vi "test wait for alive.vi"() -> ()   [LabVIEW 2014]
uses:
  user.lib/_NEVSTOP/Communicable State Machine(CSM)/_Support/Priority Queue/Priority Queue.lvclass/Priority Queue.ctl
  user.lib/_NEVSTOP/Communicable State Machine(CSM)/Utility/uuid.vi
  user.lib/_NEVSTOP/Communicable State Machine(CSM)/_Support/Process/CSMP-Async Call.vi
  user.lib/_NEVSTOP/Communicable State Machine(CSM)/Utility/Trim Both Whitespace.vi
  user.lib/_NEVSTOP/Communicable State Machine(CSM)/_Support/CSMQ/_CSMObj-Message Check.vi
  user.lib/_NEVSTOP/Communicable State Machine(CSM)/_Support/CSMQ/_CSMObj-Enqueue Cross-Module Message.vi
  user.lib/_NEVSTOP/Communicable State Machine(CSM)/_Support/CSMQ/_CSMOFGV Get.vi
  user.lib/_NEVSTOP/Communicable State Machine(CSM)/_Support/Priority Queue/Enqueue Element.vi
  user.lib/_NEVSTOP/Communicable State Machine(CSM)/Utility/Build Error Cluster.vi
  user.lib/_NEVSTOP/Communicable State Machine(CSM)/_Support/CSMQ/_CSMOFGV.vi
  user.lib/_NEVSTOP/Communicable State Machine(CSM)/Communicable State Machine.lvlib
panel:
  out "waited(ms) 2":u32
  out "waited(ms)":u32
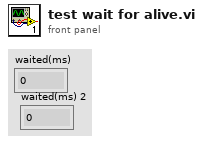
[diagram p1: front panel]
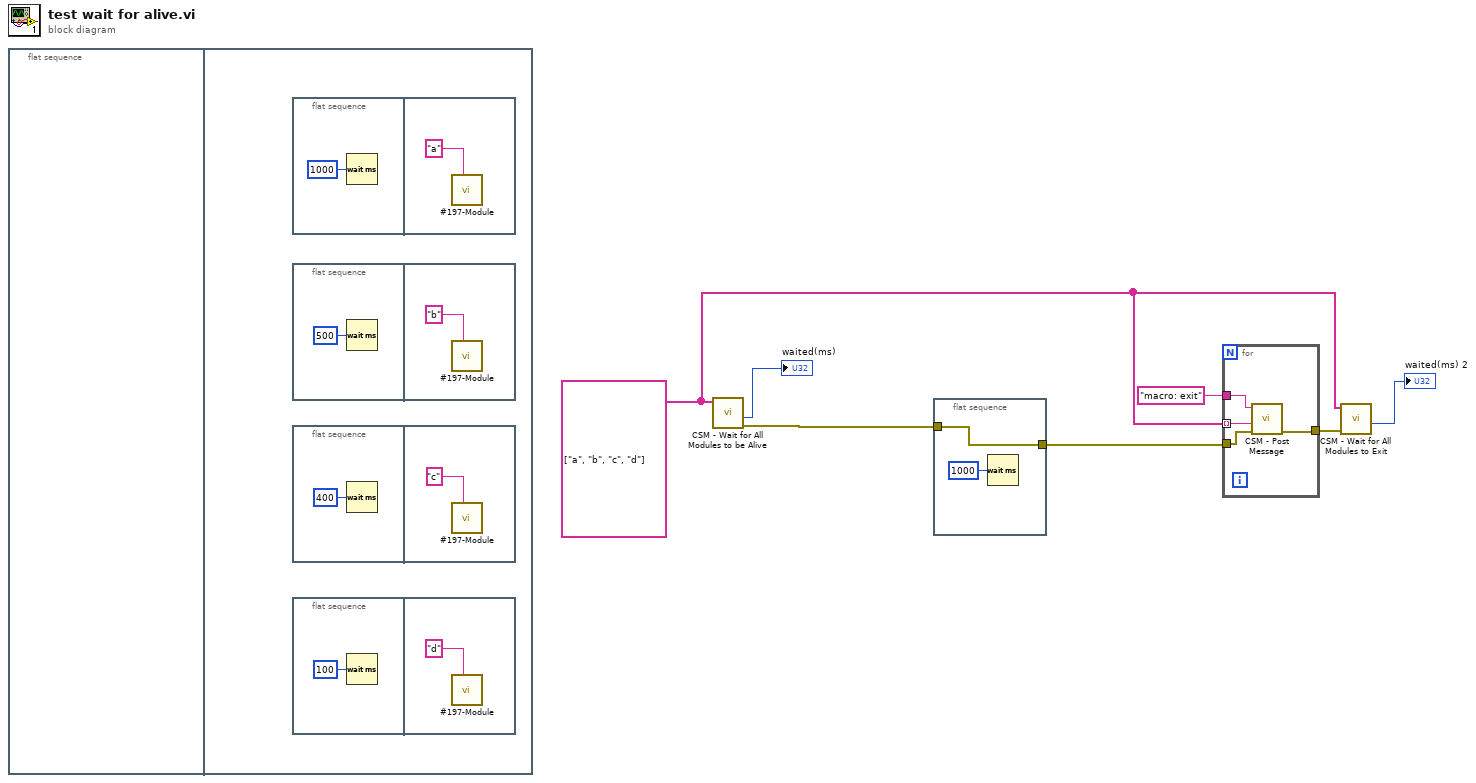
[diagram p0: block diagram]
diagram:
  w4 = string[] ["a", "b", "c", "d"] ("Module Names (in)")
  n1 = flat-sequence {
    frame #0 {
    }
    frame #1 {
      n2 = flat-sequence {
        frame #0 {
          n3 = Wait (ms)(milliseconds to wait=u32 1000) -> ()  [unwired: 1 out]
        }
        frame #1 {
          n4 = call "#197-Module.vi"("Name(\"\" to use uuid)"="a" ("Name(\"\" to use uuid)")) -> ()  [unwired: 11 in]
        }
      }
      n5 = flat-sequence {
        frame #0 {
          n6 = Wait (ms)(milliseconds to wait=u32 500) -> ()  [unwired: 1 out]
        }
        frame #1 {
          n7 = call "#197-Module.vi"("Name(\"\" to use uuid)"="b" ("Name(\"\" to use uuid)")) -> ()  [unwired: 11 in]
        }
      }
      n8 = flat-sequence {
        frame #0 {
          n9 = Wait (ms)(milliseconds to wait=u32 400) -> ()  [unwired: 1 out]
        }
        frame #1 {
          n10 = call "#197-Module.vi"("Name(\"\" to use uuid)"="c" ("Name(\"\" to use uuid)")) -> ()  [unwired: 11 in]
        }
      }
      n11 = flat-sequence {
        frame #0 {
          n12 = Wait (ms)(milliseconds to wait=u32 100) -> ()  [unwired: 1 out]
        }
        frame #1 {
          n13 = call "#197-Module.vi"("Name(\"\" to use uuid)"="d" ("Name(\"\" to use uuid)")) -> ()  [unwired: 11 in]
        }
      }
    }
  }
  n14 = call "CSM - Wait for All Modules to be Alive.vi"("Module Names (in)"=w4) -> ("Error out"=w1:errorcluster, "waited(ms)"=→"waited(ms)":u32)  [unwired: 8 in, 1 out]
  n15 = flat-sequence {
    tunnel: [w16] -> w2
    tunnel: w1 -> [w16]
    frame #0 {
      n16 = Wait (ms)(milliseconds to wait=u32 1000) -> ()  [unwired: 1 out]
    }
  }
  n17 = for {
    tunnel: w4 -> [w21] mode=indexing
    tunnel: "macro: exit" ("State") -> [w20]
    tunnel: [w19] -> w5
    tunnel: w2 -> [w18]
    n18 = call "CSM - Post Message.vi"("Error In (no error)"=w18, "Target Module"=w21, "State"=w20) -> ("error out"=w19:errorcluster)  [unwired: 8 in]
  }
  n19 = call "CSM - Wait for All Modules to Exit.vi"("Error in"=w5, "Module Names (in)"=w4) -> ("waited(ms)"=→"waited(ms) 2":u32)  [unwired: 7 in, 2 out]
